vi "Count by Status.vi"(10 "Status":T1, 11 "Test Case Result In":T2) -> (2 "Count":i32, 3 "Test Case Result Out":T2)   [LabVIEW 2020, in "Test Case Result.lvlib"]
uses:
  Test Case Result.lvlib
  Test Case Result.ctl
  Method Result/Method Result.ctl
  Rewrite Project/Result/Status.ctl
  Assertion Result/Assertion Result.ctl
  Assertion Result/Public/TypeDefs/Assertion Type.ctl
  Assertion Result/Public/TypeDefs/Status.ctl
  Assertion Result/Assertion Result.lvlib
  Method Result/Method Result.lvlib
  Rewrite Project/Result/Result.lvlib
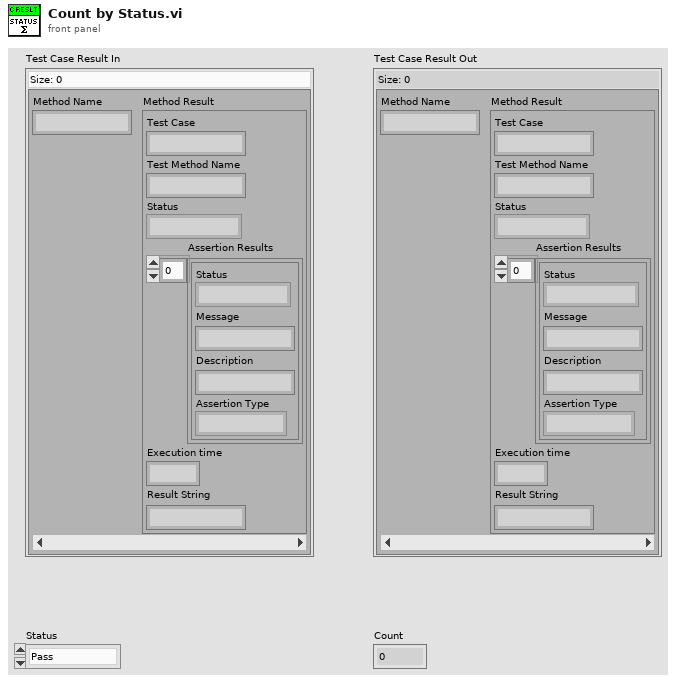
[diagram p1: front panel]
types:
  T1 = typedef "Assertion Result.lvlib/Status.ctl" = enum16{"Pass", "Fail", "Error", "Skipped", "Setup Error", "Broken", "Teardown Error"}
  T2 = typedef "Test Case Result.lvlib/Test Case Result.ctl" = map{string, T3}
  T3 = typedef "Method Result.lvlib/Method Result.ctl" = cluster{"Test Case":string, "Test Method Name":string, "Status":T4, "Assertion Results":T5[], "Execution time":dbl, "Result String":string}
  T4 = typedef "Result.lvlib/Status.ctl" = enum16{"Pass", "Fail", "Error", "Skipped", "Setup Error", "Broken", "Teardown Error"}
  T5 = typedef "Assertion Result.lvlib/Assertion Result.ctl" = cluster{"Status":T4, "Message":string, "Description":string, "Assertion Type":T6}
  T6 = typedef "Result.lvlib/Assertion Type.ctl" = enum16{"None", "Pass", "Fail", "Skip", "Pass if Equal", "Fail if Equal", "Pass if Error", "Fail if Error", "Pass if", "Fail if"}
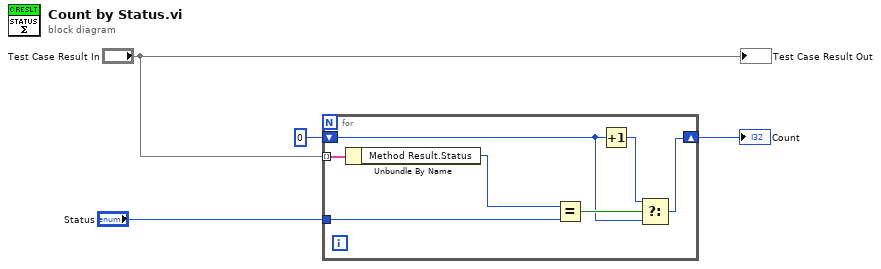
[diagram p0: block diagram]
diagram:
  n1 = for {
    tunnel: "Test Case Result In" -> [w5] mode=indexing
    shift-right: [w8] -> w3
    shift-left: 0 -> [w9]
    tunnel: "Status" -> [w7]
    n2 = Unbundle By Name(w5) -> ("Method Result.Status"=w6:T4)
    n3 = Equal?(x=w6, y=w7) -> (x = y?=w11:bool)
    n4 = Increment(x=w9) -> (x+1=w10:i32)
    n5 = Select(t=w10, s=w11, f=w9) -> (s? t:f=w8:i32)
  }
  "Count" <- w3
  "Test Case Result Out" <- "Test Case Result In"
